vi "PPS Init.vi"(8 "error in (no error)":errorcluster, 10 "VISA resource name":refnum<visa-resource-name>, 11 "IT-M6018C in":refnum<class "IT-M6018C.lvclass">) -> (0 "error out":errorcluster, 3 "IT-M6018C out":refnum<class "IT-M6018C.lvclass">)   [LabVIEW 2023, in "HardwareAbstractionLayer_LVOOP.lvlib" / "IT-M6018C.lvclass"]
uses:
  IT-M6018C.lvclass
  PowerSupply.lvclass
  <instrlib>/IT6000C/IT6000C.lvlib
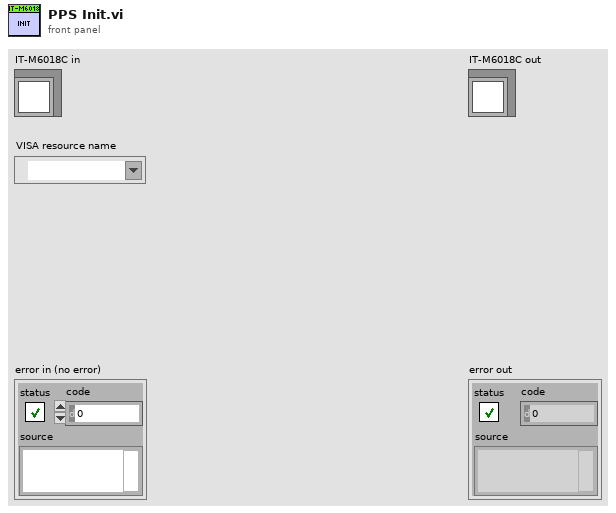
[diagram p1: front panel]
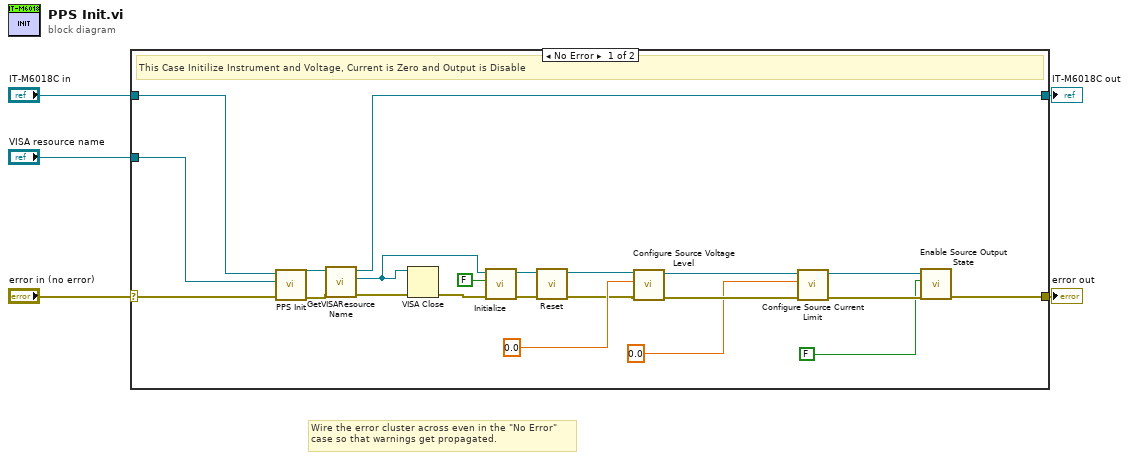
[diagram p0: block diagram]
diagram:
  # "Wire the error cluster across even in the \"No Error\"\ncase so that warnings get propagated."
  n1 = case shown="No Error" "error in (no error)" {
    selector: "error in (no error)" -> [w25 w29]
    tunnel: [w17 w29] -> w4
    tunnel: [w22 w28] -> w2
    tunnel: "IT-M6018C in" -> [w27 w28]
    tunnel: "VISA resource name" -> [w26 _]
    frame No Error {
      # "This Case Initilize Instrument and Voltage, Current is Zero and Output is Disable"
      n2 = call-parent "PPS Init.vi"("error in (no error)"=w25, "VISA resource name"=w26, "PowerSupply in"=w27) -> ("error out"=w23:errorcluster, "PowerSupply out"=w24:refnum<class "IT-M6018C.lvclass">)  [unwired: 7 in]
      n3 = call "GetVISAResourceName.vi"("error in (no error)"=w23, "object in"=w24) -> ("error out"=w7:errorcluster, "VISA resource name"=w8:refnum<visa-resource-name>, "object out"=w22:refnum<class "IT-M6018C.lvclass">)  [unwired: 7 in]
      n4 = VISA Close(VISA resource name=w8, error in (no error)=w7) -> (error out=w6:errorcluster)
      n5 = call <instrlib>:"Initialize.vi"("error in (no error)"=w6, "ID Query (True)"=FALSE, "VISA resource name"=w8) -> ("error out"=w10:errorcluster, "VISA resource name out"=w16:refnum<visa-resource-name>)  [unwired: 7 in]
      n6 = call <instrlib>:"Reset.vi"("error in (no error)"=w10, "VISA resource name"=w16) -> ("error out"=w9:errorcluster, "VISA resource name out"=w11:refnum<visa-resource-name>)  [unwired: 8 in]
      n7 = call <instrlib>:"Configure Source Voltage Level.vi"("error in (no error)"=w9, "Value(0)"=0.0, "VISA resource name"=w11) -> ("error out"=w20:errorcluster, "VISA resource name out"=w21:refnum<visa-resource-name>)  [unwired: 7 in]
      n8 = call <instrlib>:"Configure Source Current Limit.vi"("error in (no error)"=w20, "Value(0)"=0.0, "VISA resource name"=w21) -> ("error out"=w18:errorcluster, "VISA resource name out"=w19:refnum<visa-resource-name>)  [unwired: 7 in]
      n9 = call <instrlib>:"Enable Source Output State.vi"("error in (no error)"=w18, "Enable(True)"=FALSE, "VISA resource name"=w19) -> ("error out"=w17:errorcluster)  [unwired: 7 in, 1 out]
    }
    frame Error {
    }
  }
  "error out" <- w4
  "IT-M6018C out" <- w2
